vi "PRIME Detector Parse String inside Quotes.vi"(11 "Quoted String":string) -> (3 "Contents of Quotes":string)   [LabVIEW 2024, in "PRIME Detector.lvclass"]
uses:
  PRIME Detector.lvclass
  <vilib>/regexp/Match Regular Expression.xnode
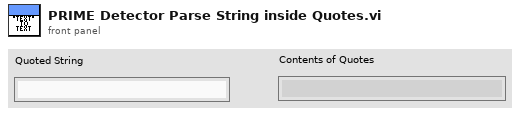
[diagram p1: front panel]
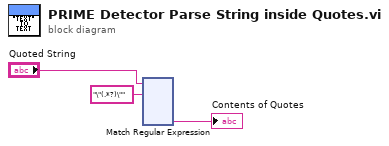
[diagram p0: block diagram]
diagram:
  n1 = xnode "Match Regular Expression"("input string"="Quoted String", "regular expression"="\"(.*?)\"") -> ("submatch 1"=→"Contents of Quotes":string)  [unwired: 4 in, 5 out]
